vi "Create All Message Queues.vi"(8 "error in (no error)":errorcluster, 11 "Process Name":string) -> (0 "error out":errorcluster, 3 "Message Queues":T1)   [LabVIEW 2018, in "TCU Module.lvlib"]
uses:
  TCU Module.lvlib
  All Message Queues.ctl
  support/Message Queue/Message Cluster.ctl
  Config Module/Controls/OP Window Display.ctl
  TCU Module Display.ctl
  support/Message Queue/Enqueue Message (Single).vi
  support/Message Queue/Message Queue.lvlib
  Feed Module/Feed Module.lvlib
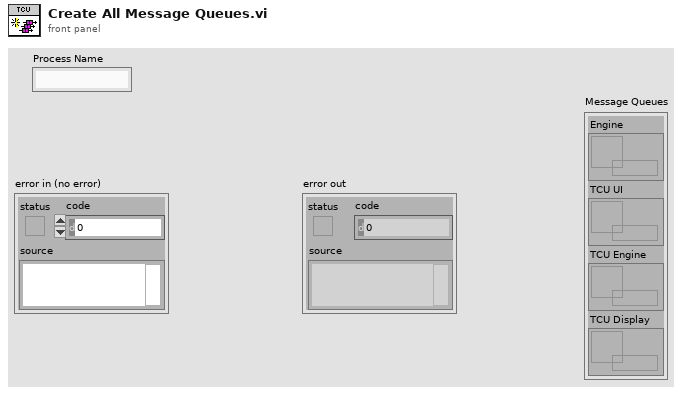
[diagram p1: front panel]
types:
  T1 = typedef "TCU Module.lvlib/All Message Queues.ctl" = cluster{"Engine":refnum<queue>, "TCU UI":refnum<queue>, "TCU Engine":refnum<queue>, "TCU Display":refnum<queue>}
  T2 = typedef "TCU Module.lvlib/TCU Module Display.ctl" = cluster{"TCU On?":bool, "Cycle Period":dbl, "Current TCU Temp":dbl}
  T3 = typedef "Feed Module.lvlib/OP Window Display.ctl" = cluster{"Flow":dbl, "Manual":dbl, "Pump Status":u16}
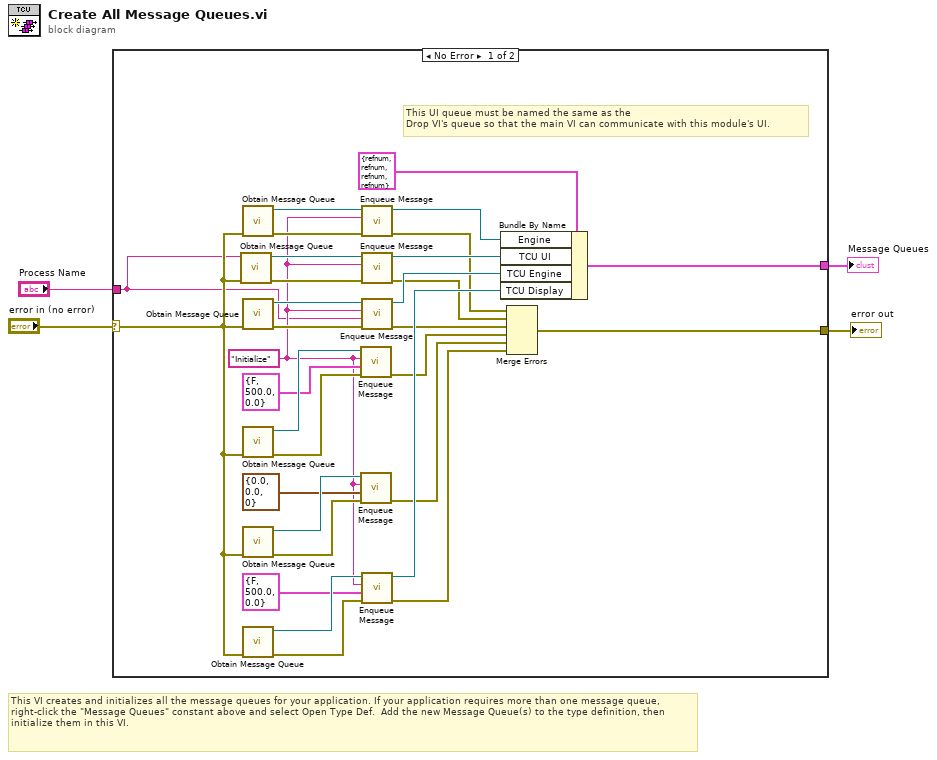
[diagram p0: block diagram]
diagram:
  # "This VI creates and initializes all the message queues for your application. If your application requires more than one message queue, right-click the \"Message Queues\" constant above and select Open Type Def.  Add the new Message Queue(s) to the type definition, then initialize them in this VI."
  n1 = case shown="No Error" "error in (no error)" {
    selector: "error in (no error)" -> [w15 w36]
    tunnel: [w34 w36] -> w4
    tunnel: [w35 _] -> w2
    tunnel: "Process Name" -> [w5 _]
    frame No Error {
      w10 = "Initialize" ("Message")
      # "This UI queue must be named the same as the \nDrop VI's queue so that the main VI can communicate with this module's UI."
      n2 = call "Obtain Message Queue.vi"("error in (no error)"=w15, "name (unnamed)"=w5) -> ("error out"=w16:errorcluster, "Message Queue"=w25:refnum<queue>)  [unwired: 8 in]
      n3 = call "Obtain Message Queue.vi"("error in (no error)"=w15) -> ("error out"=w32:errorcluster, "Message Queue"=w33:refnum<queue>)  [unwired: 9 in]
      n4 = call "Obtain Message Queue.vi"("error in (no error)"=w15) -> ("error out"=w23:errorcluster, "Message Queue"=w24:refnum<queue>)  [unwired: 9 in]
      n5 = call "Obtain Message Queue.vi"("error in (no error)"=w15) -> ("error out"=w30:errorcluster, "Message Queue"=w29:refnum<queue>)  [unwired: 9 in]
      n6 = call "Obtain Message Queue.vi"("error in (no error)"=w15) -> ("error out"=w28:errorcluster, "Message Queue"=w27:refnum<queue>)  [unwired: 9 in]
      n7 = call "Obtain Message Queue.vi"("error in (no error)"=w15) -> ("error out"=w21:errorcluster, "Message Queue"=w22:refnum<queue>)  [unwired: 9 in]
      n8 = call-poly "Enqueue Message.vi"("error in (no error)"=w30, "Message Data"=T2 {"TCU On?"=FALSE, "Cycle Period"=500.0, "Current TCU Temp"=0.0} ("PM Display"), "Message"=w10, "Message Queue"=w29) -> ("error out"=w8:errorcluster)  [unwired: 6 in, 1 out]
      n9 = call-poly "Enqueue Message.vi"("error in (no error)"=w28, "Message Data"=T3 {"Flow"=0.0, "Manual"=0.0, "Pump Status"=0}, "Message"=w10, "Message Queue"=w27) -> ("error out"=w9:errorcluster)  [unwired: 6 in, 1 out]
      n10 = call-poly "Enqueue Message.vi"("error in (no error)"=w32, "Message"=w10, "Message Queue"=w33) -> ("error out"=w11:errorcluster, "dup Message Queue"=w31:refnum<queue>)  [unwired: 7 in]
      n11 = call-poly "Enqueue Message.vi"("error in (no error)"=w16, "Message"=w10, "Message Queue"=w25) -> ("error out"=w6:errorcluster, "dup Message Queue"=w20:refnum<queue>)  [unwired: 7 in]
      n12 = call-poly "Enqueue Message.vi"("error in (no error)"=w23, "Message Data"=w5, "Message"=w10, "Message Queue"=w24) -> ("error out"=w7:errorcluster, "dup Message Queue"=w19:refnum<queue>)  [unwired: 6 in]
      n13 = call-poly "Enqueue Message.vi"("error in (no error)"=w21, "Message Data"=T2 {"TCU On?"=FALSE, "Cycle Period"=500.0, "Current TCU Temp"=0.0} ("FM Display"), "Message"=w10, "Message Queue"=w22) -> ("error out"=w17:errorcluster, "dup Message Queue"=w18:refnum<queue>)  [unwired: 6 in]
      n14 = Bundle By Name(cluster=T1 {"Engine"=refnum, "TCU UI"=refnum, "TCU Engine"=refnum, "TCU Display"=refnum} ("Message Queues"), "Engine"=w31, "TCU UI"=w20, "TCU Engine"=w19, "TCU Display"=w18) -> (w35:T1)
      n15 = Merge Errors(w11, w6, w7, w8, w9, w17) -> (w34:errorcluster)
    }
    frame Error {
    }
  }
  "Message Queues" <- w2
  "error out" <- w4
